vi "vowels const.vi"() -> ()   [LabVIEW 2019]
panel:
  out "vowel":dbl
  out "const":dbl
  in  "Input String":string
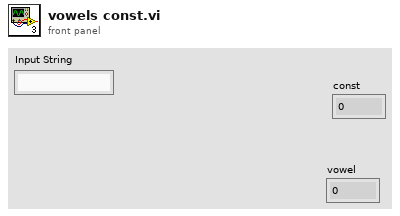
[diagram p1: front panel]
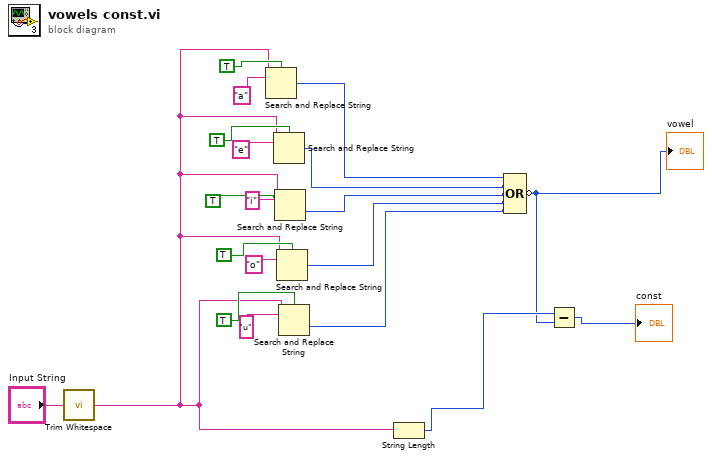
[diagram p0: block diagram]
diagram:
  n1 = call <vilib>:"Trim Whitespace.vi"("string"="Input String") -> ("trimmed string"=w3:string)  [unwired: 1 in]
  n2 = Search and Replace String(case sensitive?=TRUE, input string=w3, search string="a") -> (number of replacements=w9:i32)  [unwired: 5 in, 3 out]
  n3 = Search and Replace String(case sensitive?=TRUE, input string=w3, search string="e") -> (number of replacements=w8:i32)  [unwired: 5 in, 3 out]
  n4 = Search and Replace String(case sensitive?=TRUE, input string=w3, search string="i") -> (offset past replacement=w7:i32)  [unwired: 5 in, 3 out]
  n5 = Search and Replace String(case sensitive?=TRUE, input string=w3, search string="o") -> (number of replacements=w6:i32)  [unwired: 5 in, 3 out]
  n6 = Search and Replace String(case sensitive?=TRUE, input string=w3, search string="u") -> (offset past replacement=w5:i32)  [unwired: 5 in, 3 out]
  n7 = String Length(string=w3) -> (length=w2:i32)
  n8 = Compound Arithmetic op=OR(w9, w8, w7, w6, w5) -> (invert w1:i32)
  "vowel" <- w1
  n9 = Subtract(x=w2, y=w1) -> (x-y=→"const":i32)
